vi "数组排序.vi"(11 "数组输入":dbl[](array[numeric])) -> (3 "数组输出":dbl[](array[numeric]))   [LabVIEW 2014]
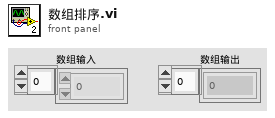
[diagram p1: front panel]
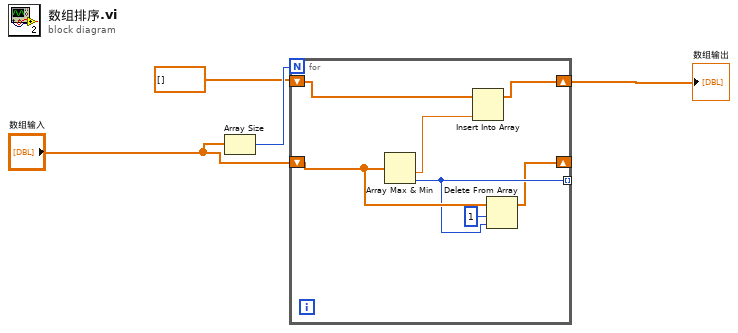
[diagram p0: block diagram]
diagram:
  n1 = Array Size(array="数组输入") -> (size(s)=w4:i32)
  n2 = for {
    N: w4 -> [_]
    tunnel: [w6] -> _ mode=indexing
    shift-right: [w10] -> w2
    shift-left: dbl[] [] -> [w11]
    shift-right: [w5] -> _
    shift-left: "数组输入" -> [w8]
    n3 = Array Max & Min(array=w8) -> (min value=w9:dbl, min index (indices)=w6:i32)  [unwired: 2 out]
    n4 = Insert Into Array(array=w11, new element=w9) -> (w10:dbl[])  [unwired: 1 in]
    n5 = Delete From Array(array=w8, length=1 ("长度"), index=w6) -> (array with subset deleted=w5:dbl[])  [unwired: 1 out]
  }
  "数组输出" <- w2
